vi "Cleanup (User).vi"(8 "error in":errorcluster, 11 "Node in":refnum<class "ThermotronDriver.lvclass">) -> (0 "error in":errorcluster, 3 "Node out":refnum<class "ThermotronDriver.lvclass">)   [LabVIEW 2023, in "ThermotronDriver.lvlib" / "ThermotronDriver.lvclass"]
uses:
  ThermotronDriver.lvclass
  ThermotronDriver.lvclass/ThermotronDriver.ctl
  Support/LabVIEW API/Thermotron8800InstrumentDriver64bitForLabView2018/Thermotron 8800/Thermotron 8800.lvlib
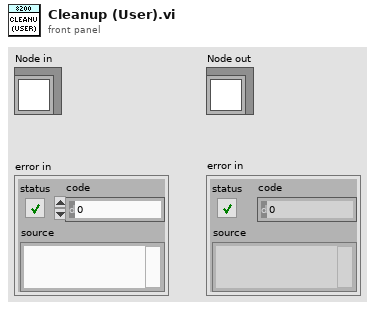
[diagram p1: front panel]
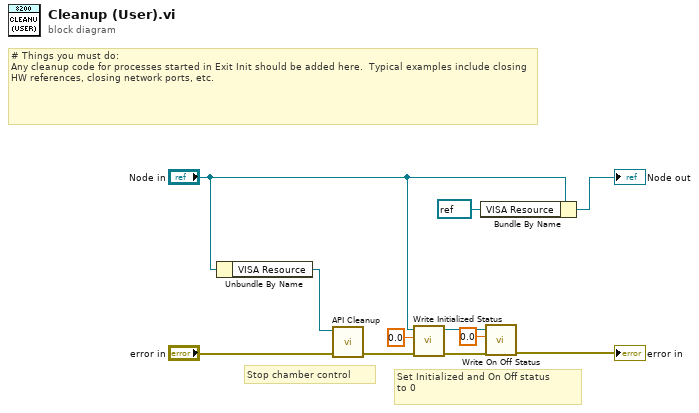
[diagram p0: block diagram]
diagram:
  # "Set Initialized and On Off status\nto 0"
  # "Stop chamber control"
  # "# Things you must do:\nAny cleanup code for processes started in Exit Init should be added here.  Typical examples include closing HW references, closing network ports, etc."
  n1 = Unbundle By Name("Node in") -> ("VISA Resource"=w10:refnum<visa-resource-name>)
  n2 = call "API Cleanup.vi"("error in"="error in", "VISA resource name"=w10) -> ("error out"=w7:errorcluster)  [unwired: 9 in]
  n3 = call-dynamic "Write Initialized Status.vi"("error in (no error)"=w7, "Initialized Status"=0.0, "ThermotronDriver in"="Node in") -> ("error out"=w4:errorcluster, "ThermotronDriver out"=w3:refnum<class "ThermotronDriver.lvclass">)  [unwired: 7 in]
  n4 = Bundle By Name(cluster="Node in", "VISA Resource"=refnum<visa-resource-name> refnum) -> (→"Node out":refnum<class "ThermotronDriver.lvclass">)
  n5 = call-dynamic "Write On Off Status.vi"("error in (no error)"=w4, "On Off Status"=0.0, "ThermotronDriver in"=w3) -> ("error out"=→"error in":errorcluster)  [unwired: 7 in, 1 out]
